vi "pmu_Create Warning MSG.vi"(6 "analog out of range":bool, 8 "error in (no error)":errorcluster, 9 "df/dt out of range":bool, 10 "freq out of range":bool, 11 "phasor out of range":bool) -> (0 "error out":errorcluster)   [LabVIEW 2014, in "NI_EP_PMU.lvlib"]
uses:
  <vilib>/addons/Electrical Power/PMU/NI_EP_PMU.lvlib
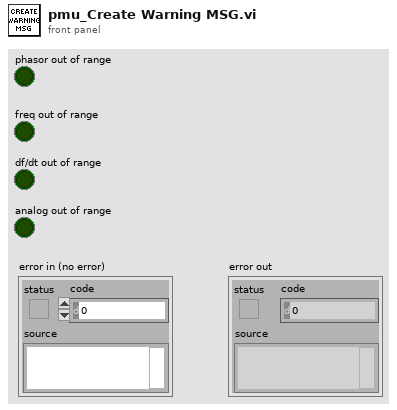
[diagram p1: front panel]
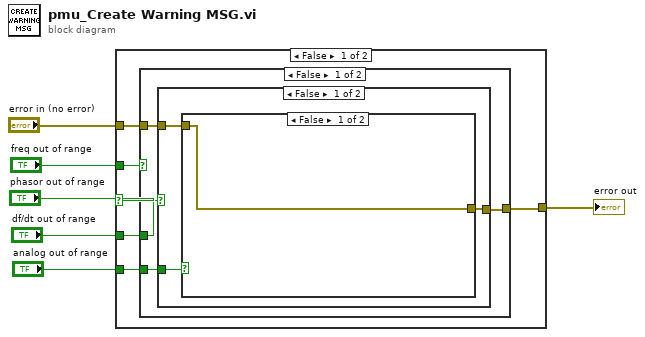
[diagram p0: block diagram]
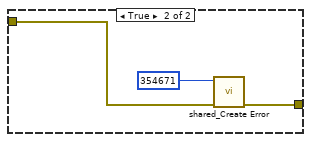
[diagram p2: hidden frame]
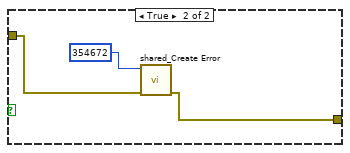
[diagram p3: hidden frame]
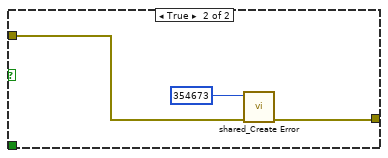
[diagram p4: hidden frame]
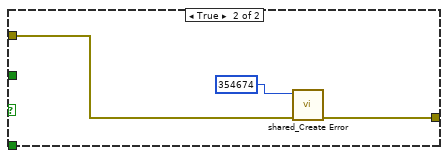
[diagram p5: hidden frame]
diagram:
  n1 = case shown="False" "phasor out of range" {
    tunnel: [w7 w31] -> w1
    tunnel: "error in (no error)" -> [w11 w30]
    tunnel: "freq out of range" -> [w10 _]
    tunnel: "df/dt out of range" -> [w9 _]
    tunnel: "analog out of range" -> [w8 _]
    frame False {
      n2 = case shown="False" w10 {
        tunnel: w11 -> [w14 w28]
        tunnel: w9 -> [w15 _]
        tunnel: w8 -> [w13 _]
        tunnel: [w12 w27] -> w7
        frame False {
          n3 = case shown="False" w15 {
            tunnel: w14 -> [w18 w25]
            tunnel: w13 -> [w17 _]
            tunnel: [w16 w23] -> w12
            frame False {
              n4 = case shown="False" w17 {
                tunnel: w18 -> [w19 w22]
                tunnel: [w19 w20] -> w16
                frame False {
                }
                frame True {
                  n5 = call <vilib>:"shared_Create Error.vi"("error in (no error)"=w22, "error code (0)"=354671 ("code")) -> ("error out"=w20:errorcluster)  [unwired: 9 in]
                }
              }
            }
            frame True {
              n6 = call <vilib>:"shared_Create Error.vi"("error in (no error)"=w25, "error code (0)"=354672 ("code")) -> ("error out"=w23:errorcluster)  [unwired: 9 in]
            }
          }
        }
        frame True {
          n7 = call <vilib>:"shared_Create Error.vi"("error in (no error)"=w28, "error code (0)"=354673 ("code")) -> ("error out"=w27:errorcluster)  [unwired: 9 in]
        }
      }
    }
    frame True {
      n8 = call <vilib>:"shared_Create Error.vi"("error in (no error)"=w30, "error code (0)"=354674 ("code")) -> ("error out"=w31:errorcluster)  [unwired: 9 in]
    }
  }
  "error out" <- w1
